vi "ExtTrig GUI.vi"() -> ()   [LabVIEW 2014]
uses:
  <vilib>/DAQmx/create/channels.llb/DAQmx Create Channel (AO-Voltage-Basic).vi
  <vilib>/DAQmx/configure/timing.llb/DAQmx Timing (Sample Clock).vi
  <vilib>/DAQmx/write.llb/DAQmx Write (Analog 1D DBL 1Chan NSamp).vi
  <vilib>/Utility/error.llb/Error Cluster From Error Code.vi
  <vilib>/rvi/errors/niLvFpgaAdjustHostInterfaceError.vi
  <vilib>/FPGAPlugInAG/PXI-7854R/niLvFpga_Close_PXI-7854R.vi
  <vilib>/rvi/interface/nirviMethod/nirviMethod.xnode
  FPGA Bitfiles/ExtTrigAugerFPGA_FPGATarget_ExtTrigAuger_gh1ysR8M8Js.lvbitx
  FPGA vi/ExtTrigAuger.vi
  <vilib>/rvi/interface/nirviCloseFPGA/nirviCloseFPGA.xnode
  <vilib>/rvi/errors/niLvFpgaMergeErrorWithErrorCode.vi
  <vilib>/FPGAPlugInAG/PXI-7854R/niLvFpga_ReadFifo_PXI-7854R.vi
panel:
  in  "FIFO depth":u32=8000
  out "FIFO transfers":u32
  out "period":dbl format="%_3p"
  in  "output size":i32=10000
  out "DAC error out":errorcluster
  in  "rate":dbl=1000.0 format="%.3p"
  out "trigger time":sgl format="%_4p"
  out "trigger count":u32
  out "FIFO Depth":u32
  in  "stop":bool
  out "FPGA error":errorcluster
  out "loop count":i32
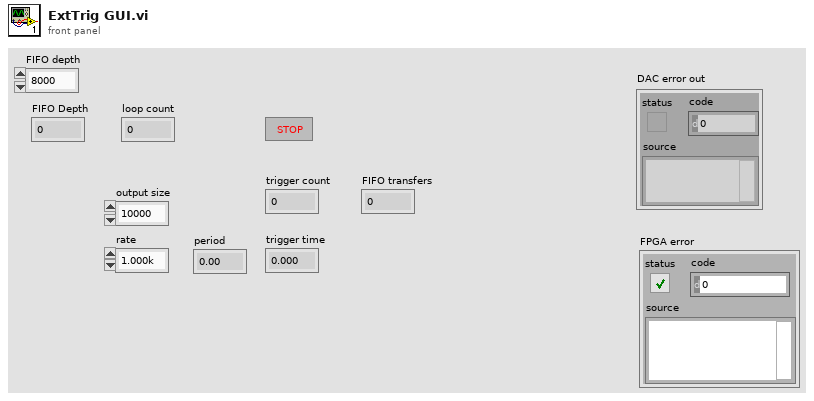
[diagram p1: front panel]
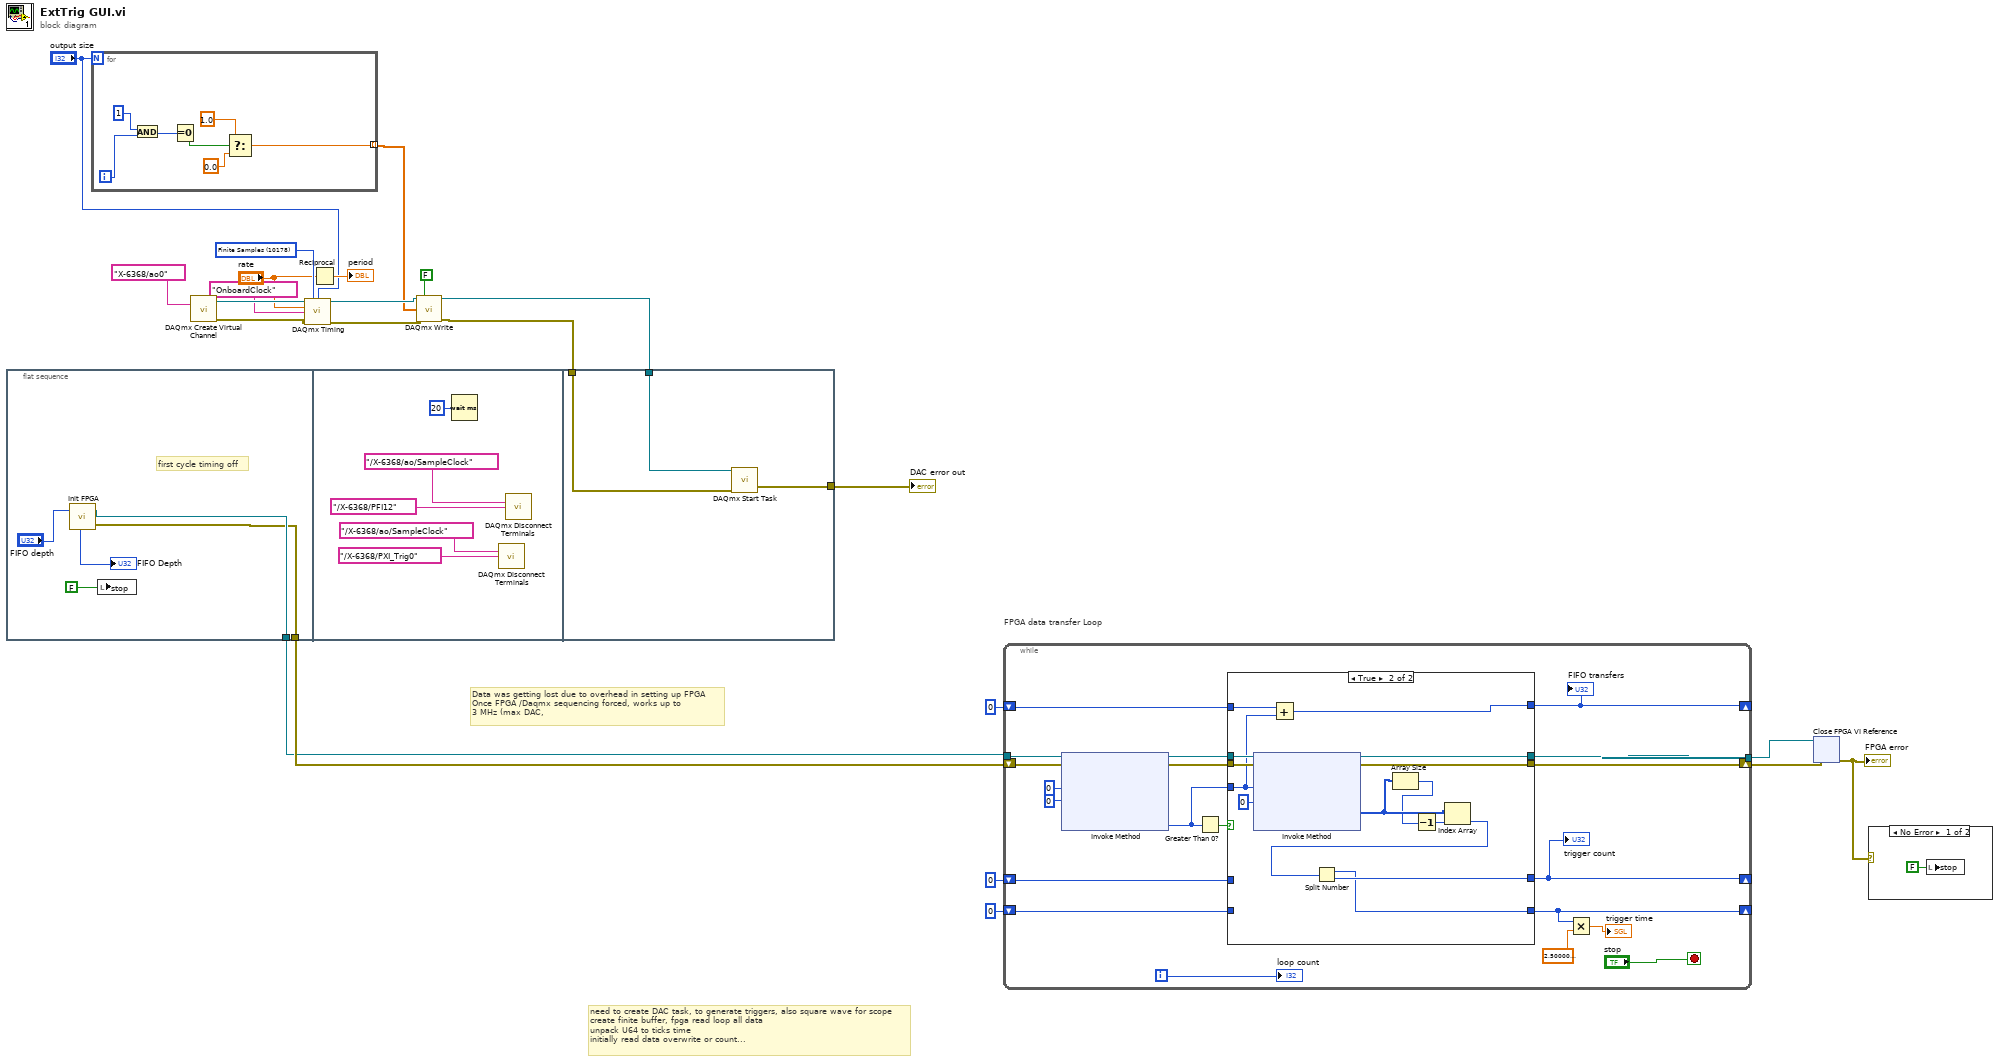
[diagram p0: block diagram]
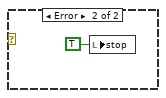
[diagram p2: hidden frame]
diagram:
  w10 = 10178 items=["Finite Samples"=10178, "Continuous Samples"=10123, "Hardware Timed Single Point"=12522] ("sample mode")
  # "Data was getting lost due to overhead in setting up FPGA\nOnce FPGA /Daqmx sequencing forced, works up to \n3 MHz (max DAC,"
  # "need to create DAC task, to generate triggers, also square wave for scope\ncreate finite buffer, fpga read loop all data\nunpack U64 to ticks time\ninitially read data overwrite or count..."
  n1 = flat-sequence {
    tunnel: [w24] -> w5
    tunnel: [w25] -> w4
    tunnel: [w36] -> w3
    tunnel: w2 -> [w35]
    tunnel: w1 -> [w34]
    frame #0 {
      # "first cycle timing off"
      n2 = call "Init FPGA.vi"("FIFO depth"="FIFO depth") -> ("FPGA error out"=w24:errorcluster, "FPGA VI Reference Out"=w25:refnum<k20>, "Actual Depth"=→"FIFO Depth":u32)
      n3 = local write "stop"(FALSE ("stop")) -> ()
    }
    frame #1 {
      n4 = Wait (ms)(milliseconds to wait=u32 20) -> ()  [unwired: 1 out]
      n5 = call <vilib>:"DAQmx Disconnect Terminals.vi"("source terminal"=tag "/X-6368/ao/SampleClock", "destination terminal"=tag "/X-6368/PXI_Trig0") -> ()  [unwired: 13 in, 1 out]
      n6 = call <vilib>:"DAQmx Disconnect Terminals.vi"("source terminal"=tag "/X-6368/ao/SampleClock", "destination terminal"=tag "/X-6368/PFI12") -> ()  [unwired: 13 in, 1 out]
    }
    frame #2 {
      n7 = call <vilib>:"DAQmx Start Task.vi"("task/channels in"=w34, "error in"=w35) -> ("error out"=w36:errorcluster)  [unwired: 12 in, 1 out]
    }
  }
  n8 = for {
    N: "output size" -> [_]
    tunnel: [w41] -> w13 mode=indexing
    i -> [w40]
    n9 = And(x=1, y=w40) -> (x .and. y?=w37:i32)
    n10 = Equal To 0?(x=w37) -> (x = 0?=w38:bool)
    n11 = Select(t=1.0, s=w38, f=0.0) -> (s? t:f=w41:dbl)
  }
  n12 = call-poly <vilib>:"DAQmx Create Virtual Channel.vi"("physical channels"=tag "X-6368/ao0") -> ("task out"=w17:refnum<k21>, "error out"=w15:errorcluster)  [unwired: 13 in]
  n13 = call-poly <vilib>:"DAQmx Timing.vi"("task/channels in"=w17, "sample mode"=w10, "samples per channel"="output size", "rate"="rate", "source"=tag "OnboardClock", "error in"=w15) -> ("task out"=w16:refnum<k21>, "error out"=w14:errorcluster)  [unwired: 8 in]
  n14 = Reciprocal(x="rate") -> (1/x=→"period":dbl)
  n15 = call-poly <vilib>:"DAQmx Write.vi"("task/channels in"=w16, "auto start"=FALSE, "data"=w13, "error in"=w14) -> ("task out"=w1:refnum<k21>, "error out"=w2:errorcluster)  [unwired: 9 in, 1 out]
  n16 = while "FPGA data transfer Loop" {
    tunnel: w4 -> [w63]
    shift-right: [w46] -> w23
    shift-left: w5 -> [w62]
    tunnel: [w45] -> w22
    shift-right: [w54] -> _
    shift-left: u32 0 -> [w53]
    shift-right: [w51] -> _
    shift-left: u32 0 -> [w52]
    shift-right: [w47] -> _
    shift-left: u32 0 -> [w48]
    i -> [w61]
    stop <- "stop" stop-if-true
    n17 = xnode "Invoke Method"("FPGA VI Reference In"=w63, "error in"=w62, "Number of Elements"=u32 0, "Timeout (ms)"=0) -> ("FPGA VI Reference Out"=w58:refnum<k20>, "error out"=w57:errorcluster, "Elements Remaining"=w56:u32)  [unwired: 1 out]
    n18 = Greater Than 0?(x=w56) -> (x > 0?=w55:bool)
    n19 = case shown="True" w55 {
      tunnel: w58 -> [w68 w82]
      tunnel: w57 -> [w67 w81]
      tunnel: w56 -> [_ w72]
      tunnel: [w68 w79] -> w45
      tunnel: [w67 w78] -> w46
      tunnel: [w66 w75] -> w54
      tunnel: w53 -> [w66 _]
      tunnel: w52 -> [w65 _]
      tunnel: [w65 w74] -> w51
      tunnel: w48 -> [w64 w73]
      tunnel: [w64 w71] -> w47
      frame False {
      }
      frame True {
        n20 = xnode "Invoke Method"("FPGA VI Reference In"=w82, "error in"=w81, "Number of Elements"=w72, "Timeout (ms)"=0) -> ("FPGA VI Reference Out"=w79:refnum<k20>, "error out"=w78:errorcluster, "Data"=w77:u64[])  [unwired: 1 out]
        n21 = Add(x=w73, y=w72) -> (x+y=w71:u32)
        n22 = Array Size(array=w77) -> (size(s)=w69:i32)
        n23 = Decrement(x=w69) -> (x-1=w70:i32)
        n24 = Index Array(array=w77, index=w70) -> (element=w76:u64)
        n25 = Split Number(x=w76) -> (hi(x)=w74:u32, lo(x)=w75:u32)
      }
    }
    "trigger count" <- w54
    "FIFO transfers" <- w47
    n26 = Multiply(x=w51, y=sgl 2.5e-08) -> (x*y=→"trigger time":sgl)
    "loop count" <- w61
  }
  n27 = xnode "Close FPGA VI Reference"("FPGA VI Reference In"=w22, "error in"=w23) -> ("error out"=w21:errorcluster)
  "FPGA error" <- w21
  n28 = case shown="No Error" w21 {
    frame No Error {
      n29 = local write "stop"(FALSE ("stop")) -> ()
    }
    frame Error {
      (unwired) FALSE ("stop")
      (unwired) FALSE ("stop")
      (unwired) FALSE ("stop")
      n30 = local write "stop"(TRUE ("stop")) -> ()
    }
  }
  "DAC error out" <- w3
